vi "LivePosition.vi"() -> ()   [LabVIEW 2015]
uses:
  <vilib>/Platform/TimedLoop/XDataNode/timing_clust.ctl
  <vilib>/Platform/TimedLoop/XDataNode/nitl_modes.ctl
  <vilib>/Platform/TimedLoop/XDataNode/wakeup.ctl
  <vilib>/Platform/TimedLoop/XDataNode/XDataNode.xnode
  <userlib>/Newport ESP301/Newport ESP301.lvlib
  <vilib>/Platform/TimedLoop/XDataNode/XDNodeRunTimeDep.lvlib
panel:
  in  "stop 2":bool
  out "Axis 3 Pos.":dbl
  out "Axis 2 Pos.":dbl
  out "Axis 1 Pos.":dbl
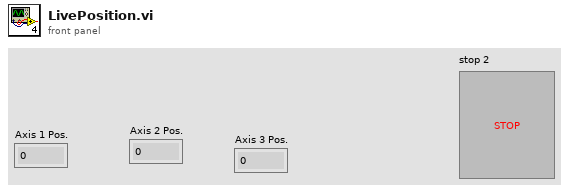
[diagram p1: front panel]
types:
  T1 = typedef "XDNodeRunTimeDep.lvlib/timing_clust.ctl" = cluster{"Expected End [f-1]":u64, "Actual End [f-1]":u64, "Finished Late? [f-1]":bool, "Expected End [i-1]":u64, "Actual End [i-1]":u64, "Finished Late? [i-1]":bool, "Expected Start [i]":u64, "Actual Start [i]":u64, "Expected Start [f]":u64, "Actual Start [f]":u64, "Source Name":string, "Structure Name":string, "Period":i64, "Deadline":i64, "Offset":i64, "Start":i64, "Priority":i32, "Timeout":i32, "Mode":T2, "Wakeup Reason":T3, "Error":errorcluster, "Source Type":string, "Secondary Source Type":string, "Global End Time":u64, "Global Start Time":u64, "Frame Duration":u64, "Iteration Duration":u64, "Assigned CPU":i32, "I/O Scan Engine Mode":u32}
  T2 = typedef "XDNodeRunTimeDep.lvlib/nitl_modes.ctl" = enum32{"No Change", "Process missed periods, maintain original phase", "Discard missed periods, maintain original phase", "Process missed periods, ignore original phase", "Discard missed periods, ignore original phase"}
  T3 = typedef "XDNodeRunTimeDep.lvlib/wakeup.ctl" = enum32{"Normal", "Aborted", "Asynchronous wakeup", "Timing source error", "Timed loop error", "Timeout"}
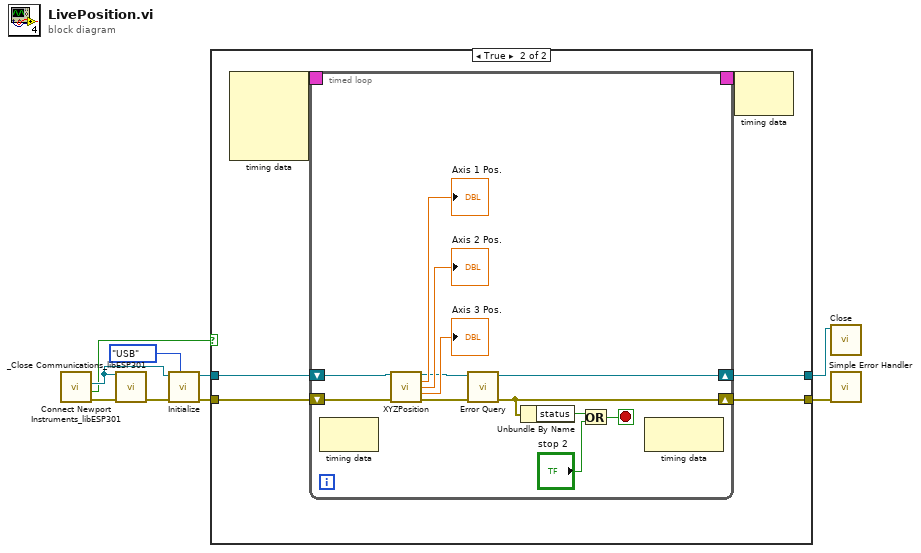
[diagram p0: block diagram]
diagram:
  n1 = call <userlib>:"Connect Newport Instruments_libESP301.vi"() -> ("error (duplicate)"=w7:errorcluster, "Connected"=w4:bool, "VISA resource name (duplicate)"=w6:refnum<visa-resource-name>)  [unwired: 7 in, 2 out]
  n2 = call <userlib>:"_Close Communications_libESP301.vi"("Instrument Channel"=w6, "error in (no error)"=w7) -> ("error out"=w9:errorcluster)  [unwired: 13 in]
  n3 = call <userlib>:"Initialize.vi"("VISA resource name"=w6, "error in (no error)"=w9, "Serial Link (USB)"=enum16{"RS232", "USB"}."USB" ("Serial Link (RS232)")) -> ("VISA resource name out"=w5:refnum<visa-resource-name>, "error out"=w3:errorcluster)  [unwired: 6 in]
  n4 = case shown="True" w4 {
    tunnel: [w11 w17] -> w2
    tunnel: [w10 w16] -> w1
    tunnel: w5 -> [w11 w15]
    tunnel: w3 -> [w10 w14]
    frame False {
    }
    frame True {
      n5 = node-c288() -> (w13:T1)  [unwired: 4 in]
      n6 = timed-loop {
        timing: w13 -> [_]
        timing-out: [_] -> w12
        shift-right: [w22] -> w17
        shift-left: w15 -> [w26]
        shift-right: [w20] -> w16
        shift-left: w14 -> [w25]
        stop <- w18 stop-if-true
        n7 = node-c288() -> ()  [unwired: 1 in, 1 out]
        n8 = call "XYZPosition.vi"("VISA resource name"=w26, "error in"=w25) -> ("VISA resource name out"=w23:refnum<visa-resource-name>, "Axis 1"=→"Axis 1 Pos.":dbl, "Axis 2"=→"Axis 2 Pos.":dbl, "Axis 3"=→"Axis 3 Pos.":dbl, "error out"=w24:errorcluster)  [unwired: 9 in]
        n9 = call <userlib>:"Error Query.vi"("error in (no error)"=w24, "VISA resource name"=w23) -> ("error out"=w20:errorcluster, "VISA resource name out"=w22:refnum<visa-resource-name>)  [unwired: 2 in, 2 out]
        n10 = Unbundle By Name(w20) -> ("status"=w19:bool)
        n11 = Or(x=w19, y="stop 2") -> (x .or. y?=w18:bool)
        n12 = node-c288() -> ()  [unwired: 1 in, 1 out]
      }
      n13 = node-c288(w12) -> ()  [unwired: 1 out]
    }
  }
  n14 = call <userlib>:"Close.vi"("VISA resource name"=w2) -> ()  [unwired: 10 in, 1 out]
  n15 = call <vilib>:"Simple Error Handler.vi"("error in (no error)"=w1) -> ()  [unwired: 1 in, 8 out]
